vi "Plot.vi"(0 "ToneCloud in":refnum<class "Tone Cloud.lvclass">, 7 "action":string="init", 11 "error in (no error)":errorcluster) -> (4 "ToneCloud out":refnum<class "Tone Cloud.lvclass">, 15 "error out":errorcluster)   [LabVIEW 2015, in "Tone Cloud.lvclass"]
uses:
  Tone Cloud.lvclass
  Tone Cloud.lvclass/Tone Cloud.ctl
  Utility VIs/Math VIs/LinSpace (start-stop-step).vi
panel:
  out "colorbar":picture
  in  "Freq axis":dbl(slide) caption="Amplitude" scale=0.0..44.0
  out "Graph":cluster{"Graph":dbl[], "Graph":dbl[]}[](graph)
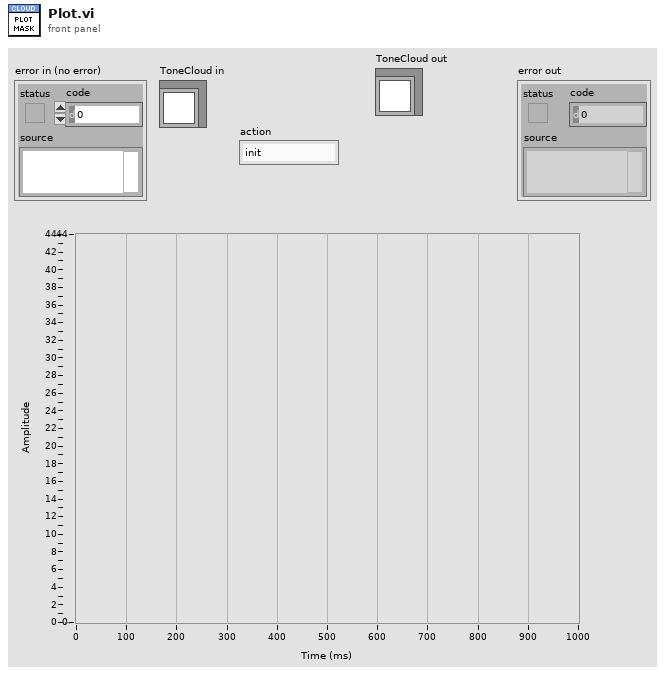
[diagram p1: front panel]
types:
  T1 = enum16{"User", "Prism", "Kelly", "Dark2", "Sequential", "Hue"}
  T2 = typedef "LVRectTypeDef.ctl" = cluster{"Left":i16, "Top":i16, "Right":i16, "Bottom":i16}
  T3 = typedef "LVPoint32TypeDef.ctl" = cluster{"Horizontal":i32, "Vertical":i32}
  T4 = cluster{"Horizontal":i32, "Vertical":i32, "Horizontal":i32, "Vertical":i32}
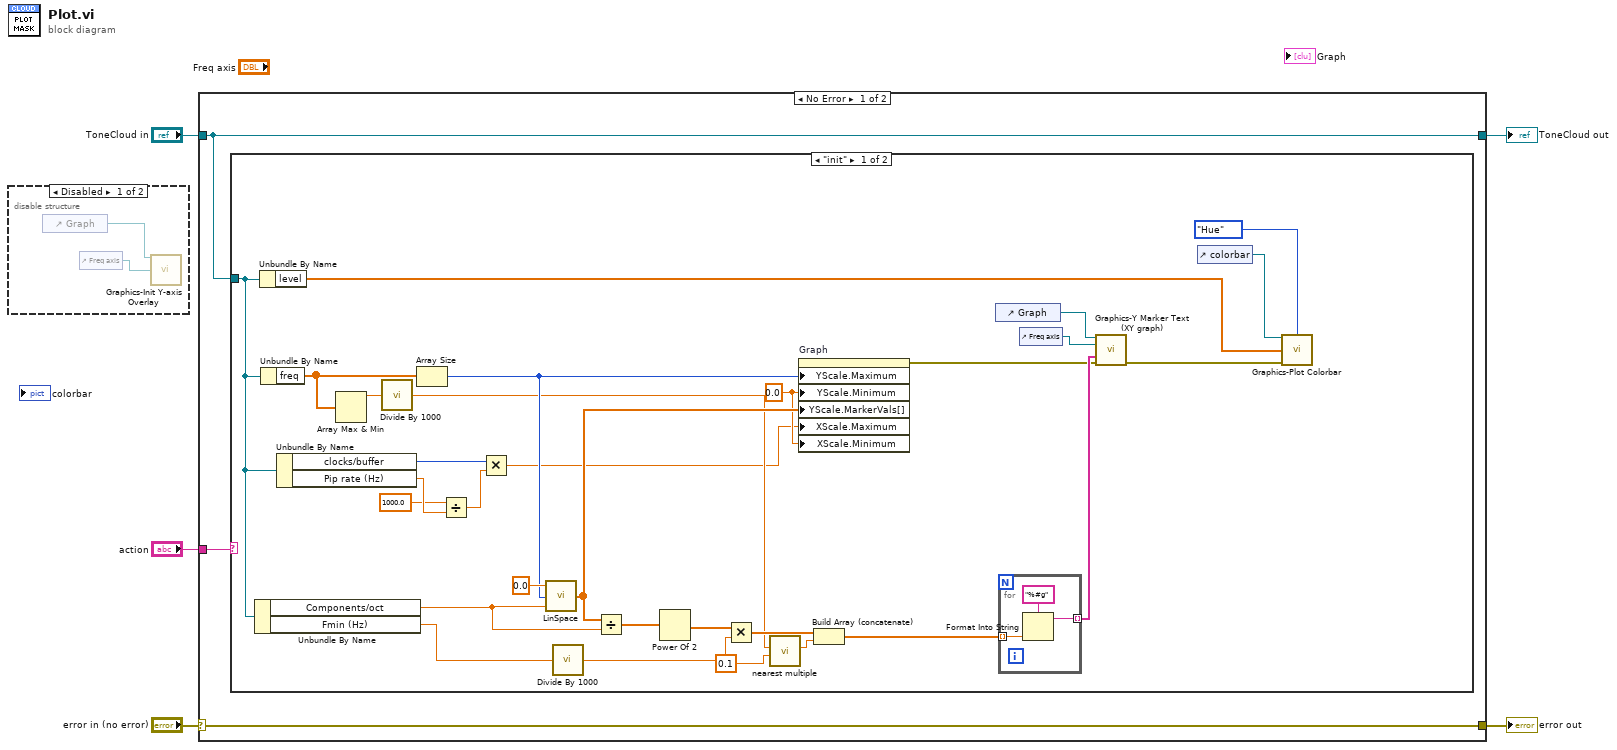
[diagram p0: block diagram]
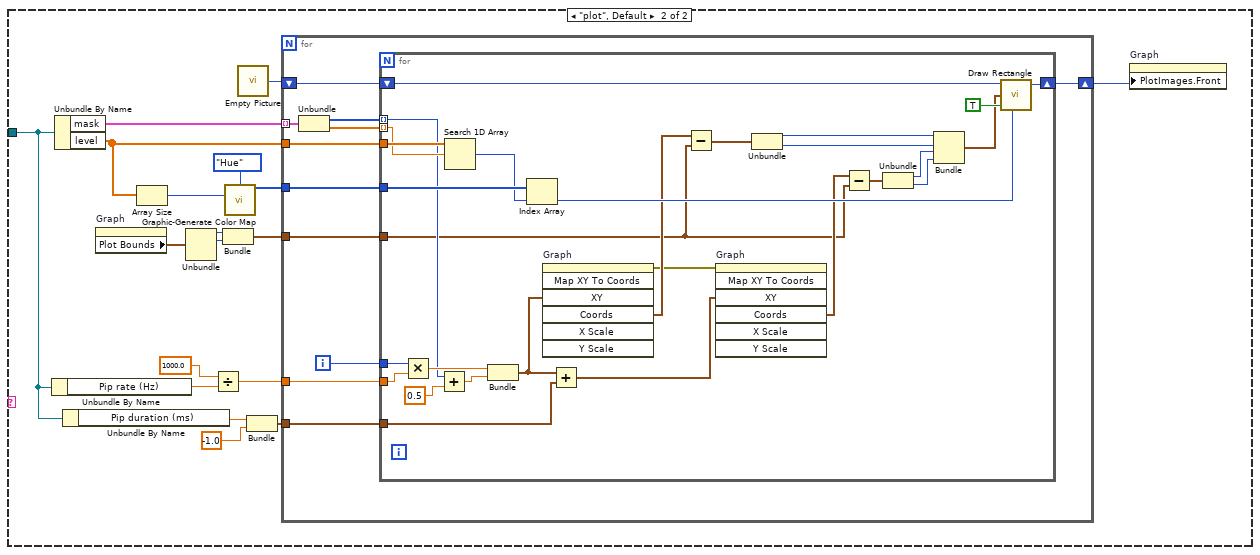
[diagram p3: hidden frame]
diagram:
  n1 = disable-structure shown="Disabled" {
    frame Disabled {
      n2 = control-ref of="Graph"() -> (w7:refnum<vi>)
      n3 = control-ref of="Freq axis"() -> (w6:refnum<vi>)
      n4 = call "Graphics-Init Y-axis Overlay.vi"("Ctl Refnum"=w7, "Y-axis slider"=w6) -> ()  [unwired: 13 in, 1 out]
    }
    frame Enabled {
    }
  }
  n5 = case shown="No Error" "error in (no error)" {
    selector: "error in (no error)" -> [w8 w102]
    tunnel: [w8 w102] -> w4
    tunnel: [w10 w101] -> w2
    tunnel: "ToneCloud in" -> [w10 w101]
    tunnel: "action" -> [w9 _]
    frame No Error {
      n6 = case shown="\"init\"" w9 {
        tunnel: w10 -> [w15 w47]
        frame "init" {
          w21 = 0.0 ("Y Scale.Range:Minimum")
          n7 = Unbundle By Name(w15) -> ("Components/oct"=w39:dbl, "Fmin (Hz)"=w36:dbl)
          n8 = Unbundle By Name(w15) -> ("level"=w12:dbl[])
          n9 = Unbundle By Name(w15) -> ("freq"=w30:dbl[])
          n10 = Unbundle By Name(w15) -> ("clocks/buffer"=w16:i32, "Pip rate (Hz)"=w20:dbl)
          n11 = Array Max & Min(array=w30) -> (max value=w29:dbl)  [unwired: 3 out]
          n12 = call "Divide By 1000.vi"("X"=w29) -> ("X/1000"=w26:dbl)
          n13 = Array Size(array=w30) -> (size(s)=w33:i32)
          n14 = Divide(x=1000.0, y=w20) -> (x/y=w18:dbl)
          n15 = Multiply(x=w16, y=w18) -> (x*y=w17:dbl)
          n16 = call-poly "LinSpace.vi"("Step"=w39, "Stop"=w33, "Start"=0.0 ("Y Scale.Range:Minimum")) -> ("Array"=w32:dbl[])  [unwired: 1 in, 1 out]
          n17 = call "Divide By 1000.vi"("X"=w36) -> ("X/1000"=w35:dbl)
          n18 = Divide(x=w32, y=w39) -> (x/y=w38:dbl[])
          n19 = Power Of 2(x=w38) -> (2^x=w37:dbl[])
          n20 = Multiply(x=w37, y=w35) -> (x*y=w34:dbl[])
          n21 = call "nearest multiple.vi"("y"=0.1, "x"=w26) -> ("round(x/y)*y"=w28:dbl)  [unwired: 7 in, 2 out]
          n22 = property on="Graph" class="XYGraph (strict)"("YScale.Maximum"=w33, "YScale.Minimum"=w21, "YScale.MarkerVals[]"=w32, "XScale.Maximum"=w17, "XScale.Minimum"=w21) -> (error out=w22:errorcluster)  [unwired: 2 in, 1 out]
          n23 = Build Array (concatenate)(w34, w28) -> (w31:dbl[])
          n24 = control-ref of="Graph"() -> (w25:refnum<vi>)
          n25 = for {
            tunnel: w31 -> [w43] mode=indexing
            tunnel: [w42] -> w23 mode=indexing
            n26 = Format Into String(format string="%#g" ("initial string"), w43) -> (resulting string=w42:string)  [unwired: 2 in, 1 out]
          }
          n27 = control-ref of="Freq axis"() -> (w24:refnum<vi>)
          n28 = call "Graphics-Y Marker Text (XY graph).vi"("Graph"=w25, "Slider"=w24, "Text Labels[]"=w23, "error in (no error)"=w22) -> ("error out"=w14:errorcluster)  [unwired: 11 in]
          n29 = control-ref of="colorbar"() -> (w13:refnum<vi>)
          n30 = call "Graphics-Plot Colorbar.vi"("Picture in"=w13, "Map"=T1."Hue", "Values"=w12, "error in (no error)"=w14) -> ()  [unwired: 11 in, 1 out]
        }
        frame "plot", Default {
          n31 = Unbundle By Name(w47) -> ("Pip rate (Hz)"=w50:dbl)
          n32 = Unbundle By Name(w47) -> ("mask"=w61:cluster{"index":i32[], "level":dbl[]}[], "level"=w56:dbl[])
          n33 = Unbundle By Name(w47) -> ("Pip duration (ms)"=w46:dbl)
          n34 = property on="Graph" class="XYGraph (strict)"() -> ("Plot Bounds"=w52:T2)  [unwired: 2 in, 2 out]
          n35 = Array Size(array=w56) -> (size(s)=w58:i32)
          n36 = Unbundle(w52) -> ("Left"=w55:i16, "Top"=w53:i16)  [unwired: 2 out]
          n37 = Divide(x=1000.0, y=w50) -> (x/y=w48:dbl)
          n38 = Bundle("Left"=w55, "Top"=w53) -> (w54:cluster{"Left":i16, "Top":i16})  [unwired: 1 in]
          n39 = call "Graphic-Generate Color Map.vi"("Map"=T1."Hue", "Size"=w58) -> ("Colors"=w57:u32[])  [unwired: 13 in]
          n40 = call "Empty Picture"() -> ("empty picture"=w60:picture)
          n41 = Bundle("Pip duration (ms)"=w46, -1.0) -> (w44:cluster{"Pip duration (ms)":dbl, dbl})  [unwired: 1 in]
          n42 = for {
            tunnel: w61 -> [w72] mode=indexing
            shift-right: [w69] -> w51
            shift-left: w60 -> [w68]
            tunnel: w57 -> [w67]
            tunnel: w56 -> [w66]
            tunnel: w54 -> [w64]
            tunnel: w48 -> [w63]
            tunnel: w44 -> [w62]
            i -> [w65]
            n43 = Unbundle(w72) -> ("index"=w71:i32[], "level"=w70:dbl[])
            n44 = for {
              tunnel: w71 -> [w89] mode=indexing
              tunnel: w70 -> [w97] mode=indexing
              shift-right: [w99] -> w69
              shift-left: w68 -> [w100]
              tunnel: w67 -> [w96]
              tunnel: w66 -> [w98]
              tunnel: w65 -> [w92]
              tunnel: w64 -> [w83]
              tunnel: w63 -> [w88]
              tunnel: w62 -> [w85]
              n45 = Multiply(x=w92, y=w88) -> (x*y=w91:dbl)
              n46 = Add(x=w89, y=0.5) -> (x+y=w74:dbl)
              n47 = Search 1D Array(1D array=w98, element=w97) -> (index of element=w95:i32)  [unwired: 1 in]
              n48 = Bundle(w91, w74) -> (w86:cluster{dbl, dbl})  [unwired: 1 in]
              n49 = Index Array(array=w96, index=w95) -> (element=w93:u32)
              n50 = invoke on="Graph" class="XYGraph (strict)" method="Map XY To Coords"("XY"=w86) -> (error out=w87:errorcluster, "Coords"=w90:T3)  [unwired: 6 in, 5 out]
              n51 = Add(x=w86, y=w85) -> (x+y=w75:cluster{dbl, dbl})
              n52 = Subtract(x=w90, y=w83) -> (x-y=w82:T3)
              n53 = invoke on="Graph" class="XYGraph (strict)" method="Map XY To Coords"(error in=w87, "XY"=w75) -> ("Coords"=w84:T3)  [unwired: 5 in, 6 out]
              n54 = Unbundle(w82) -> ("Horizontal"=w80:i32, "Vertical"=w79:i32)
              n55 = Subtract(x=w84, y=w83) -> (x-y=w81:T3)
              n56 = Unbundle(w81) -> ("Horizontal"=w78:i32, "Vertical"=w77:i32)
              n57 = Bundle("Horizontal"=w80, "Vertical"=w79, "Horizontal"=w78, "Vertical"=w77) -> (w76:T4)  [unwired: 1 in]
              n58 = call <vilib>:"Draw Rectangle.vi"("picture"=w100, "rect"=w76, "fill?(F)"=TRUE, "color(black)"=w93) -> ("new picture"=w99:picture)  [unwired: 5 in]
            }
          }
          n59 = property on="Graph" class="XYGraph (strict)"("PlotImages.Front"=w51) -> ()  [unwired: 2 in, 2 out]
        }
      }
    }
    frame Error {
    }
  }
  "error out" <- w4
  "ToneCloud out" <- w2
